vi "Twitter Open - Desktop.vi"(8 "error in":errorcluster, 9 "Access Credentials (in)":T1, 10 "Consumer Secret":string, 11 "Consumer Key":string) -> (0 "error out":errorcluster, 1 "Access Credentials (out)":T1, 3 "Twitter Handle Out":T2={"OAuth Credentials"={"Signature Method"=enum."HMAC-SHA1", "Version"="1.0", "Client"={"Token"="", "Secret"=""}, "Access"={"Token"="", "Secret"=""}}, "since ID"="", "max ID"="", "Screen Name"=""})   [LabVIEW 2011, in "i3-twitter.lvlib"]
doc: "<b>Twitter Open - Desktop</b> is used on Desktops with a Web Browser installed to connect to Twitter and verify that the user credentials are valid. If the user approves the application or the provided Access Credentials are valid then a Twitter Handle is returned. Applications run on platforms without Desktops or that require a specific fixed set of Access Tokens should use <b>Twitter Open - Embedded</b>.\n\nThe <b>Consumer Key</b> and <b>Consumer Secret</b> are unique to each application and can be created by making an application at dev.twitter.com. See the Twitter Getting Started Guide for more details.\n\n<b>Access Credentials</b> are created when the user runs Twitter Open and the user approves the application request. Save the Access Credentials and in the future when Twitter Open is called the Access Credentials can be provided to prevent the user from having to log in repeatedly."
uses:
  i3-twitter.lvlib
  Controls/Twitter Handle.ctl
  i3-oauth/Controls/OAuth Handle.ctl
  i3-oauth/Controls/Signature Method.ctl
  i3-oauth/Controls/Credentials.ctl
  i3-oauth/Controls/Authorization URLs.ctl
  i3-oauth/i3-oauth.lvlib
panel:
  out "Response Header":string
  out "Response Body":string
  # "Debug Only"
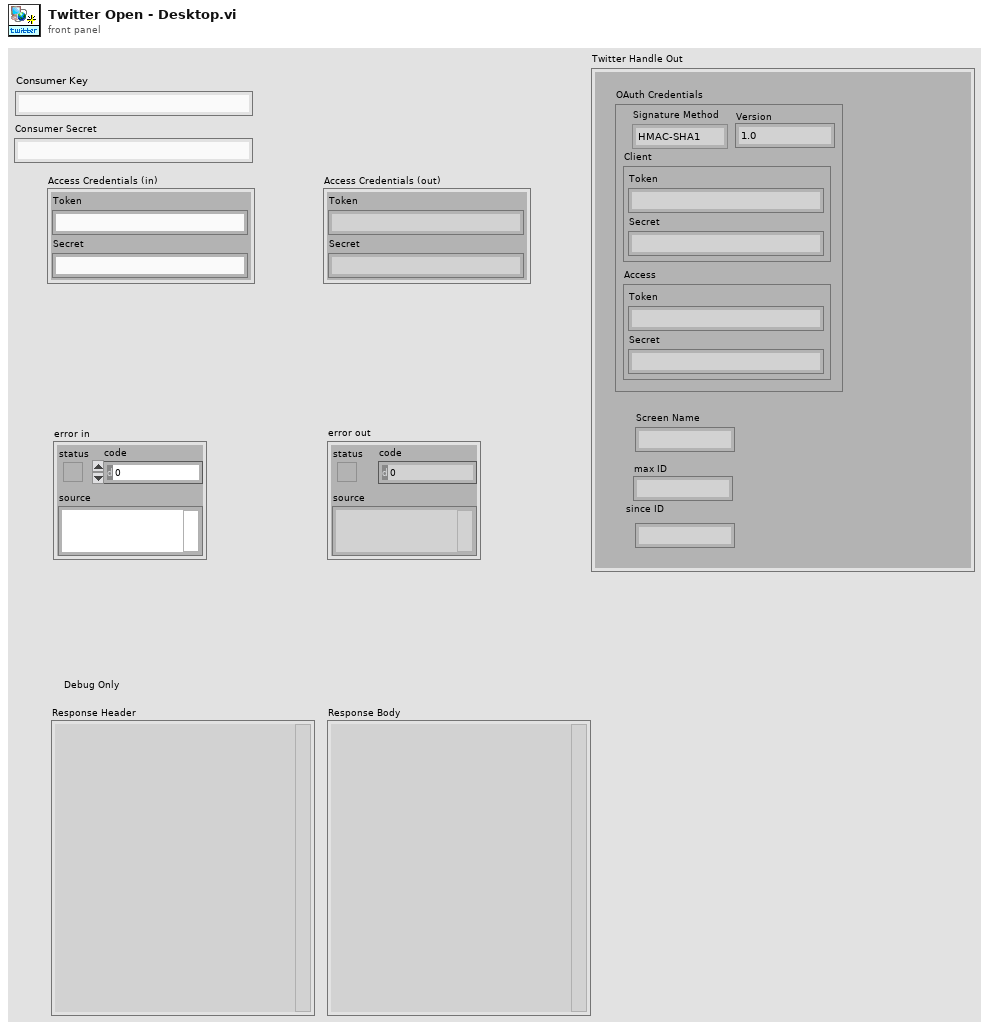
[diagram p1: front panel]
types:
  T1 = typedef "i3-oauth.lvlib/Credentials.ctl" = cluster{"Token":string, "Secret":string}
  T2 = typedef "i3-twitter.lvlib/Twitter Handle.ctl" = cluster{"OAuth Credentials":T3, "since ID":string, "max ID":string, "Screen Name":string}
  T3 = typedef "i3-oauth.lvlib/OAuth Handle.ctl" = cluster{"Signature Method":T4, "Version":string, "Client":T1, "Access":T1}
  T4 = typedef "i3-oauth.lvlib/Signature Method.ctl" = enum16{"HMAC-MD5", "HMAC-SHA1", "HMAC-SHA224", "HMAC-SHA256", "HMAC-SHA384", "HMAC-SHA512"}
  T5 = typedef "i3-oauth.lvlib/Authorization URLs.ctl" = cluster{"Request URL":string, "Authorize URL":string, "Access URL":string}
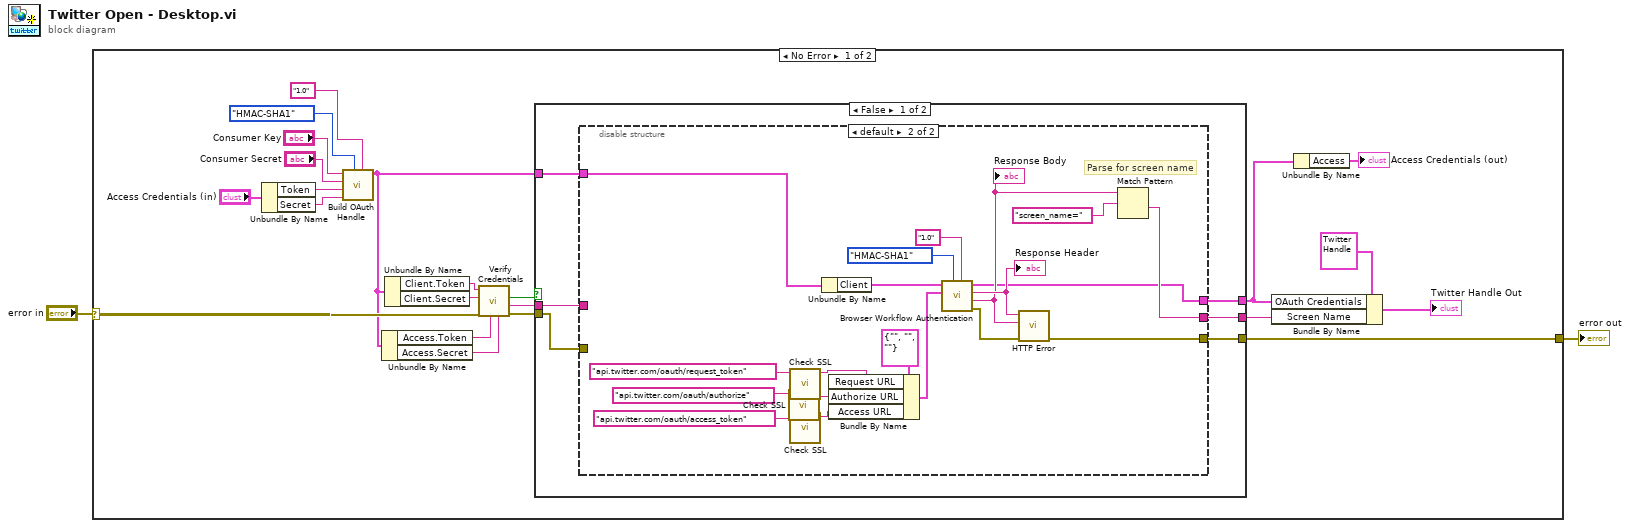
[diagram p0: block diagram]
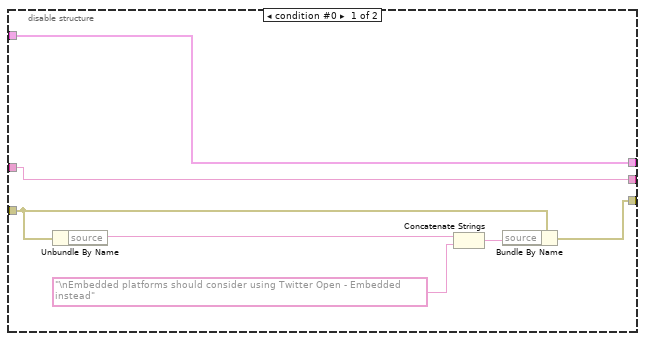
[diagram p2: hidden frame]
diagram:
  n1 = case shown="No Error" "error in" {
    selector: "error in" -> [w16 w60]
    tunnel: [w23 w60] -> w2
    frame No Error {
      n2 = Unbundle By Name("Access Credentials (in)") -> ("Token"=w11:string, "Secret"=w10:string)
      n3 = call "Build OAuth Handle.vi"("Version (1.0)"="1.0", "Signature Method (HMAC-SHA1)"=Signature_Method."HMAC-SHA1", "Access Secret"=w10, "Access Token"=w11, "Client Secret"="Consumer Secret", "Client Token"="Consumer Key") -> ("OAuth Handle"=w3:T3)  [unwired: 5 in]
      n4 = Unbundle By Name(w3) -> ("Access.Token"=w5:string, "Access.Secret"=w4:string)
      n5 = Unbundle By Name(w3) -> ("Client.Token"=w6:string, "Client.Secret"=w7:string)
      n6 = call "Verify Credentials.vi"("Access Token Secret (In)"=w4, "Access Token (In)"=w5, "error in (no error)"=w16, "Consumer Secret"=w7, "Consumer Key"=w6) -> ("error out"=w20:errorcluster, "Screen Name"=w19:string, "Success?"=w24:bool)  [unwired: 3 in, 1 out]
      n7 = case shown="False" w24 {
        tunnel: [w28 w57] -> w18
        tunnel: [w29 w59] -> w23
        tunnel: [w30 w58] -> w21
        tunnel: w20 -> [w25 w59]
        tunnel: w19 -> [w26 w58]
        tunnel: w3 -> [w27 w57]
        frame False {
          n8 = disable-structure shown="default" {
            disable-tunnel: [w36 w56] -> w30
            disable-tunnel: [w35 w54] -> w29
            disable-tunnel: [w37 w47] -> w28
            disable-tunnel: w27 -> [w37 w41]
            disable-tunnel: w26 -> [w36 _]
            disable-tunnel: w25 -> [w34 _]
            frame condition #0 {
              n9 = Unbundle By Name(w34) -> ("source"=w32:string)
              n10 = Concatenate Strings(w32, "\nEmbedded platforms should consider using Twitter Open - Embedded instead" ("string")) -> (w33:string)
              n11 = Bundle By Name(cluster=w34, "source"=w33) -> (w35:errorcluster)
            }
            frame condition #1 (active) {
              # "Parse for screen name"
              n12 = call "Check SSL.vi"("Input URL"="api.twitter.com/oauth/authorize" ("Authorize URL")) -> ("Output URL"=w44:string)  [unwired: 8 in]
              n13 = call "Check SSL.vi"("Input URL"="api.twitter.com/oauth/request_token" ("Request URL")) -> ("Output URL"=w45:string)  [unwired: 8 in]
              n14 = call "Check SSL.vi"("Input URL"="api.twitter.com/oauth/access_token" ("Access URL")) -> ("Output URL"=w43:string)  [unwired: 8 in]
              n15 = Unbundle By Name(w41) -> ("Client"=w40:T1)
              n16 = Bundle By Name(cluster=T5 {"Request URL"="", "Authorize URL"="", "Access URL"=""} ("Authorization URLs"), "Request URL"=w45, "Authorize URL"=w44, "Access URL"=w43) -> (w42:T5)
              n17 = call "Browser Workflow Authentication.vi"("Version (1.0)"="1.0", "Signature Method (HMAC-SHA1)"=Signature_Method."HMAC-SHA1", "Authorization URLs"=w42, "Client Credentials"=w40) -> ("error out"=w55:errorcluster, "Access Response Body"=w48:string, "Access Response Header"=w49:string, "OAuth Handle"=w47:T3)  [unwired: 4 in]
              "Response Body" <- w48
              "Response Header" <- w49
              n18 = call "HTTP Error.vi"("error in (no error)"=w55, "Body"=w48, "Header"=w49) -> ("error out"=w54:errorcluster)  [unwired: 6 in, 2 out]
              n19 = Match Pattern(string=w48, regular expression="screen_name=" ("format string")) -> (after substring=w56:string)  [unwired: 1 in, 3 out]
            }
          }
        }
        frame True {
        }
      }
      n20 = Bundle By Name(cluster=T2 {"OAuth Credentials"={"Signature Method"=enum."HMAC-MD5", "Version"="", "Client"={"Token"="", "Secret"=""}, "Access"={"Token"="", "Secret"=""}}, "since ID"="", "max ID"="", "Screen Name"=""} ("Twitter Handle"), "OAuth Credentials"=w18, "Screen Name"=w21) -> (→"Twitter Handle Out":T2)
      n21 = Unbundle By Name(w18) -> ("Access"=→"Access Credentials (out)":T1)
    }
    frame Error {
    }
  }
  "error out" <- w2
